vi "Image_Save_Handler.vi"(8 "Stop?":bool, 9 "Data":T2={"L16 Linear Actuator"="", "XE 1000 Pump"="", "Camera1"="", "Camera2"="", "Camera1_IMG"=refnum, "Camera2_IMG"=refnum, "Img_Capt"=FALSE, "Actuator"=FALSE, "Pump"=FALSE, "Cam 1"=FALSE, "Cam 2"=FALSE, "Empty_Refill"=FALSE, "Crop"=FALSE, "Light intensity"=100, "Exposure Time"=1000.0, "Sample Name"="Test Sample", "Operator"="MRJ", "Calibration 1"=path "C:/Users/au540322/Desktop/IHS_Project/images/Debris/Debris_0/Debris_0_2019_06_01-23-32-49-686.PNG", "Calibration 2"=path "C:/Users/au540322/Desktop/IHS_Project/images/Debris/Debris_0/Debris_0_2019_06_01-23-32-49-686.PNG", "Framerate"=1, "Timeout Sample"=0, "Collection date"="MRJ", "Sample size threshold"=1, "Empty start"=1, "Command"="MRJ", "Calibration Image 1"=refnum, "Calibration Image 2"=refnum, "Original Image 1"=refnum, "Original Image 2"=refnum, "Processing Image 1"=refnum, "Processing Image 2"=refnum, "Object Image 1"=refnum, "Object Image 2"=refnum, "Cam 1 - save queue"=refnum, "Cam 2 - save queue"=refnum, "Station"="", "Species Name"="", "Other Notes"="", "Aperture"=enum."Item 0", "Image Process Queue Size"=500, "Image Save Queue Size"=500, "Overload threshold"=500, "Max Framerate"=100, "Blue Plane Image"=refnum, "Subtract Image"=refnum, "Binary Image 1"=refnum, "ROI mask allocation"=refnum, "Rectangle 1"={"Left"=0, "Top"=0, "Right"=0, "Bottom"=0, "Rotation"=0.0}, "Rectangle 2"={"Left"=0, "Top"=0, "Right"=0, "Bottom"=0, "Rotation"=0.0}, "Binary Image 2"=refnum, "Detection Region %"=0.0, "Cam 1 queue"=refnum, "Cam 2 queue"=refnum, "Detect image 1"=refnum, "Detect image 2"=refnum, "Detect 1"=path "C:/Users/au540322/Desktop/IHS_Project/images/Debris/Debris_0/Debris_0_2019_06_01-23-32-49-686.PNG", "Detect 2"=path "C:/Users/au540322/Desktop/IHS_Project/images/Debris/Debris_0/Debris_0_2019_06_01-23-32-49-686.PNG", "Max large object threshold"=0, "Open(T)/Close(F)"=FALSE} {"Rectangle 2"."Rotation" format="%.2f"; "Rectangle 2"."Left" scale=0.0..1024.0; "Rectangle 2"."Right" scale=0.0..1024.0; "Rectangle 1"."Rotation" format="%.2f"; "Rectangle 1"."Left" scale=0.0..1024.0; "Rectangle 1"."Right" scale=0.0..1024.0; "Max Framerate" min=1; "Overload threshold" min=1; "Image Save Queue Size" min=1; "Image Process Queue Size" min=1; "Empty start" min=1; "Sample size threshold" min=1; "Framerate" min=1; "Light intensity" scale=0.0..100.0}) -> (0 "Stop out":bool, 1 "max queue":i32, 3 "Queue size":T1)   [LabVIEW 2019]
doc: "Saves image files from cameras in specified folder location."
uses:
  controls/Data.ctl
  <vilib>/userdefined/High Color/IMAQdx.ctl
  <vilib>/vision/Image Controls.llb/IMAQ Image.ctl
  Camera_ID.ctl
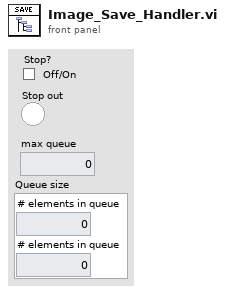
[diagram p1: front panel]
types:
  T1 = cluster{"# elements in queue":i32, "# elements in queue":i32}
  T2 = typedef "Data.ctl" = cluster{"L16 Linear Actuator":refnum<visa-resource-name>, "XE 1000 Pump":refnum<visa-resource-name>, "Camera1":T3, "Camera2":T3, "Camera1_IMG":T4, "Camera2_IMG":T4, "Img_Capt":bool, "Actuator":bool, "Pump":bool, "Cam 1":bool, "Cam 2":bool, "Empty_Refill":bool, "Crop":bool, "Light intensity":i32, "Exposure Time":dbl, "Sample Name":string, "Operator":string, "Calibration 1":path, "Calibration 2":path, "Framerate":i32, "Timeout Sample":i32, "Collection date":string, "Sample size threshold":i32, "Empty start":u32, "Command":string, "Calibration Image 1":T4, "Calibration Image 2":T4, "Original Image 1":T4, "Original Image 2":T4, "Processing Image 1":T4, "Processing Image 2":T4, "Object Image 1":T4, "Object Image 2":T4, "Cam 1 - save queue":refnum<queue>, "Cam 2 - save queue":refnum<queue>, "Station":string, "Species Name":string, "Other Notes":string, "Aperture":enum32{"Item 0", "Item 1", "Item 2", "Item 3"}, "Image Process Queue Size":i32, "Image Save Queue Size":i32, "Overload threshold":i32, "Max Framerate":i32, "Blue Plane Image":T4, "Subtract Image":T4, "Binary Image 1":T4, "ROI mask allocation":T4, "Rectangle 1":T5, "Rectangle 2":T5, "Binary Image 2":T4, "Detection Region %":dbl, "Cam 1 queue":refnum<queue>, "Cam 2 queue":refnum<queue>, "Detect image 1":T4, "Detect image 2":T4, "Detect 1":path, "Detect 2":path, "Max large object threshold":i32, "Open(T)/Close(F)":bool}
  T3 = typedef "IMAQdx.ctl" = refnum<k21>
  T4 = typedef "IMAQ Image.ctl" = refnum<image>
  T5 = typedef "IMAQ Rectangle" = cluster{"Left":i32, "Top":i32, "Right":i32, "Bottom":i32, "Rotation":dbl}
  T6 = typedef "Camera_ID.ctl" = enum16{"Camera 1", "Camera 2"}
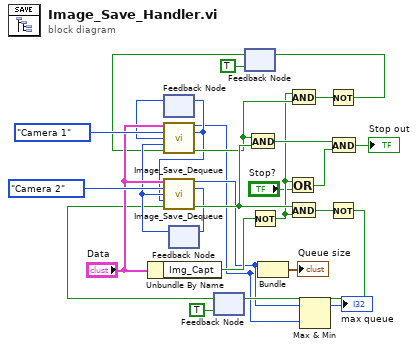
[diagram p0: block diagram]
diagram:
  n1 = Unbundle By Name("Data") -> ("Img_Capt"=w22:bool)
  n2 = feedback #1() -> (w14:i32)  [unwired: 1 in]
  n3 = feedback #2() -> (w12:i32)  [unwired: 1 in]
  n4 = feedback #3(TRUE) -> (w7:bool)
  n5 = feedback #4(TRUE) -> (w9:bool)
  n6 = call "Image_Save_Dequeue.vi"("Data"="Data", "Camera"=Camera_ID."Camera 1", "Old"=w14, "Other"=w12, "Queue active"=w9) -> ("# elements in queue"=w2:i32, "State out"=w11:i32, "Last image"=w19:bool)  [unwired: 8 in]
  n7 = feedback-in #1(w11) -> ()
  n8 = call "Image_Save_Dequeue.vi"("Data"="Data", "Camera"=Camera_ID."Camera 2", "Old"=w12, "Other"=w11, "Queue active"=w7) -> ("# elements in queue"=w3:i32, "State out"=w13:i32, "Last image"=w21:bool)  [unwired: 8 in]
  n9 = feedback-in #2(w13) -> ()
  n10 = And(x=w19, y=w21) -> (x .and. y?=w25:bool)
  n11 = Not(x=w22) -> (.not. x?=w18:bool)
  n12 = Bundle("# elements in queue"=w3, "# elements in queue"=w2) -> (→"Queue size":T1)  [unwired: 1 in]
  n13 = Or(x=w18, y="Stop?") -> (x .or. y?=w23:bool)
  n14 = And(x=w18, y=w19) -> (x .and. y?=w17:bool)
  n15 = And(x=w21, y=w18) -> (x .and. y?=w20:bool)
  n16 = Max & Min(x=w3, y=w2) -> (max(x,y)=→"max queue":i32)  [unwired: 1 out]
  n17 = Not(x=w17) -> (.not. x?=w10:bool)
  n18 = feedback-in #4(w10) -> ()
  n19 = Not(x=w20) -> (.not. x?=w8:bool)
  n20 = feedback-in #3(w8) -> ()
  n21 = And(x=w25, y=w23) -> (x .and. y?=→"Stop out":bool)
